vi "Reset Yaw.vi"(11 "To":dbl) -> ()   [LabVIEW 2015]
uses:
  Robot Global Data.vi
  navX/navX Library v2/navX Library v2.lvlib
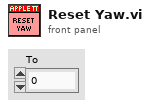
[diagram p1: front panel]
types:
  T1 = typedef "navX Library v2.lvlib/Z900_navX_DeviceTypeDef.ctl" = cluster{"Interface":cluster{"Protocol":T2, "Update Rate (4Hz-60Hz)":u8, "navX Open TypeDef":variant}, "Notify Packet":refnum<notifier>, "Loop VI Refnum":refnum<vi>, "Ready to Close Occurrence Refnum":refnum<k4>}
  T2 = typedef "navX Library v2.lvlib/Z900_navX_ProtocolTypeDef.ctl" = enum16{"SERIAL", "I2C", "SPI"}
  T3 = cluster{"Yaw":dbl, "Roll":dbl, "Pitch":dbl, "Heading":dbl, "Fused Heading":dbl}
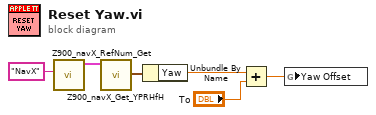
[diagram p0: block diagram]
diagram:
  n1 = call "Z900_navX_RefNum_Get.vi"("refnum name"="NavX") -> ("navX Device"=w2:T1)  [unwired: 9 in, 1 out]
  n2 = call "Z900_navX_Get_YPRHfH.vi"("navX Device"=w2) -> ("YRPHfH"=w3:T3)  [unwired: 7 in, 3 out]
  n3 = Unbundle By Name(w3) -> ("Yaw"=w1:dbl)
  n4 = Add(x=w1, y="To") -> (x+y=w6:dbl)
  n5 = global write "Robot Global Data.vi" "Yaw Offset"(w6) -> ()
